vi "黑子权值.vi"(9 "列":u8, 10 "行":dbl, 11 "当前棋盘状态":i32[][](array[numeric])) -> (3 "黑子总权值":i32)   [LabVIEW 2018]
doc: "计算当前位置对于黑子来说的权值大小。"
panel:
  out "活1?右上":bool
  out "活1?左下":bool
  out "活1?左上":bool
  out "活1?右下":bool
  out "活1?正上":bool
  out "活1?正下":bool
  out "活1?正左":bool
  out "活1?正右":bool
  out "3个黑子？右上":bool
  out "2个黑子？右上":bool
  out "1个黑子？右上":bool
  out "3个黑子？左下":bool
  out "2个黑子？左下":bool
  out "1个黑子？ 左下":bool
  out "3个黑子？左上":bool
  out "2个黑子？左上":bool
  out "1个黑子？左上":bool
  out "3个黑子？右下":bool
  out "2个黑子？右下":bool
  out "1个黑子？右下":bool
  out "3个黑子？ 正上":bool
  out "2个黑子？ 正上":bool
  out "1个黑子？ 正上":bool
  out "3个黑子？ 正下":bool
  out "2个黑子？正下":bool
  out "1个黑子？ 正下":bool
  out "3个黑子？正左":bool
  out "2个黑子？正左":bool
  out "1个黑子？正左":bool
  out "3个黑子？正右":bool
  out "2个黑子？正右":bool
  out "1个黑子？正右":bool
  out "右上方向权值":i32
  out "左下方向权值":i32
  out "左上方向权值":i32
  out "右下方向权值":i32
  out "正上方权值":i32
  out "正下方权值":i32
  out "正左方向权值":i32
  out "正右方向权值":i32
  out "前二位权值":dbl
  out "前三位权值":dbl
  # "当前\n位置"
  # "0"
  # "1"
  # "2"
  # "3"
  # "4"
  # "5"
  # "6"
  # "7"
  # "8"
  # "9"
  # "10"
  # "11"
  # "12"
  # "13"
  # "14"
  # "0"
  # "1"
  # "2"
  # "3"
  # "4"
  # "5"
  # "6"
  # "7"
  # "8"
  # "9"
  # "10"
  # "11"
  # "12"
  # "13"
  # "14"
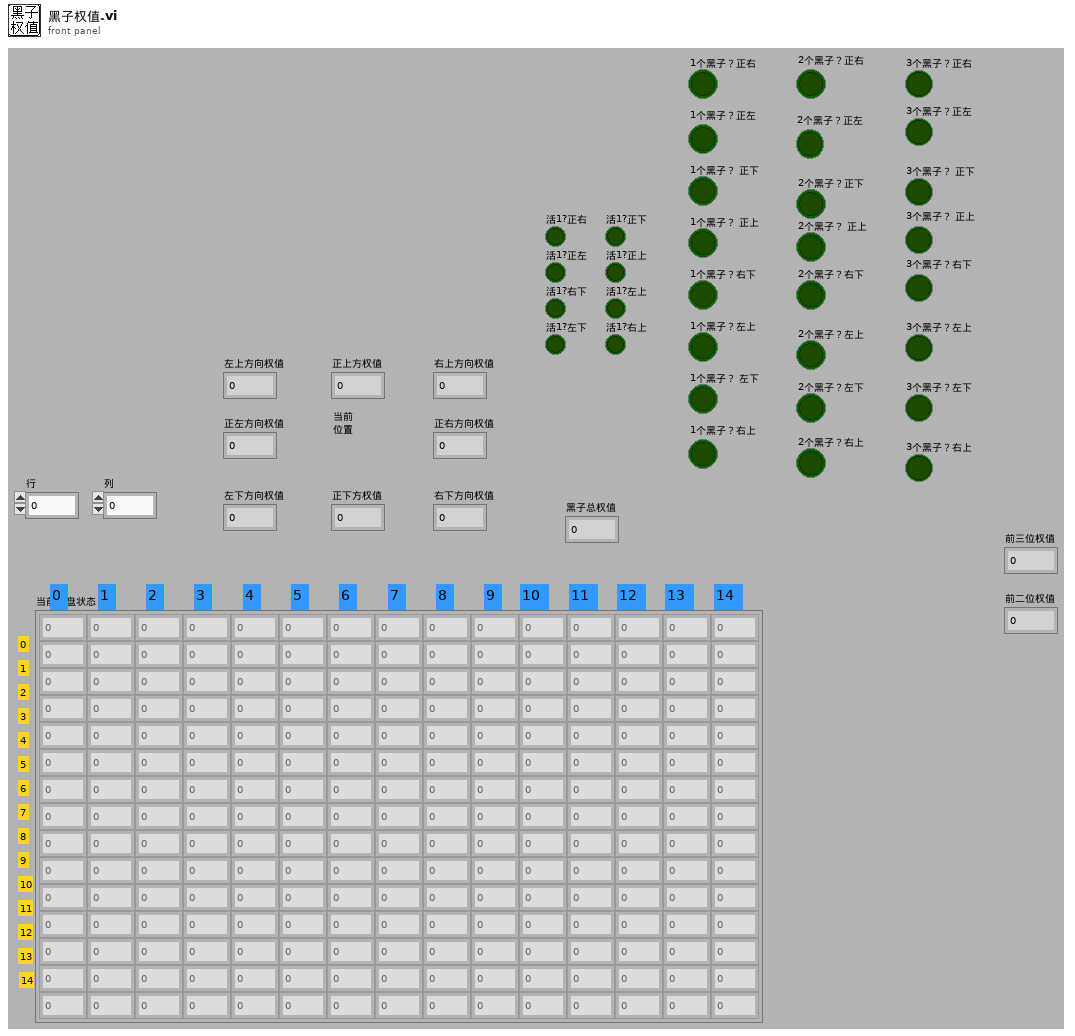
[diagram p1: front panel]
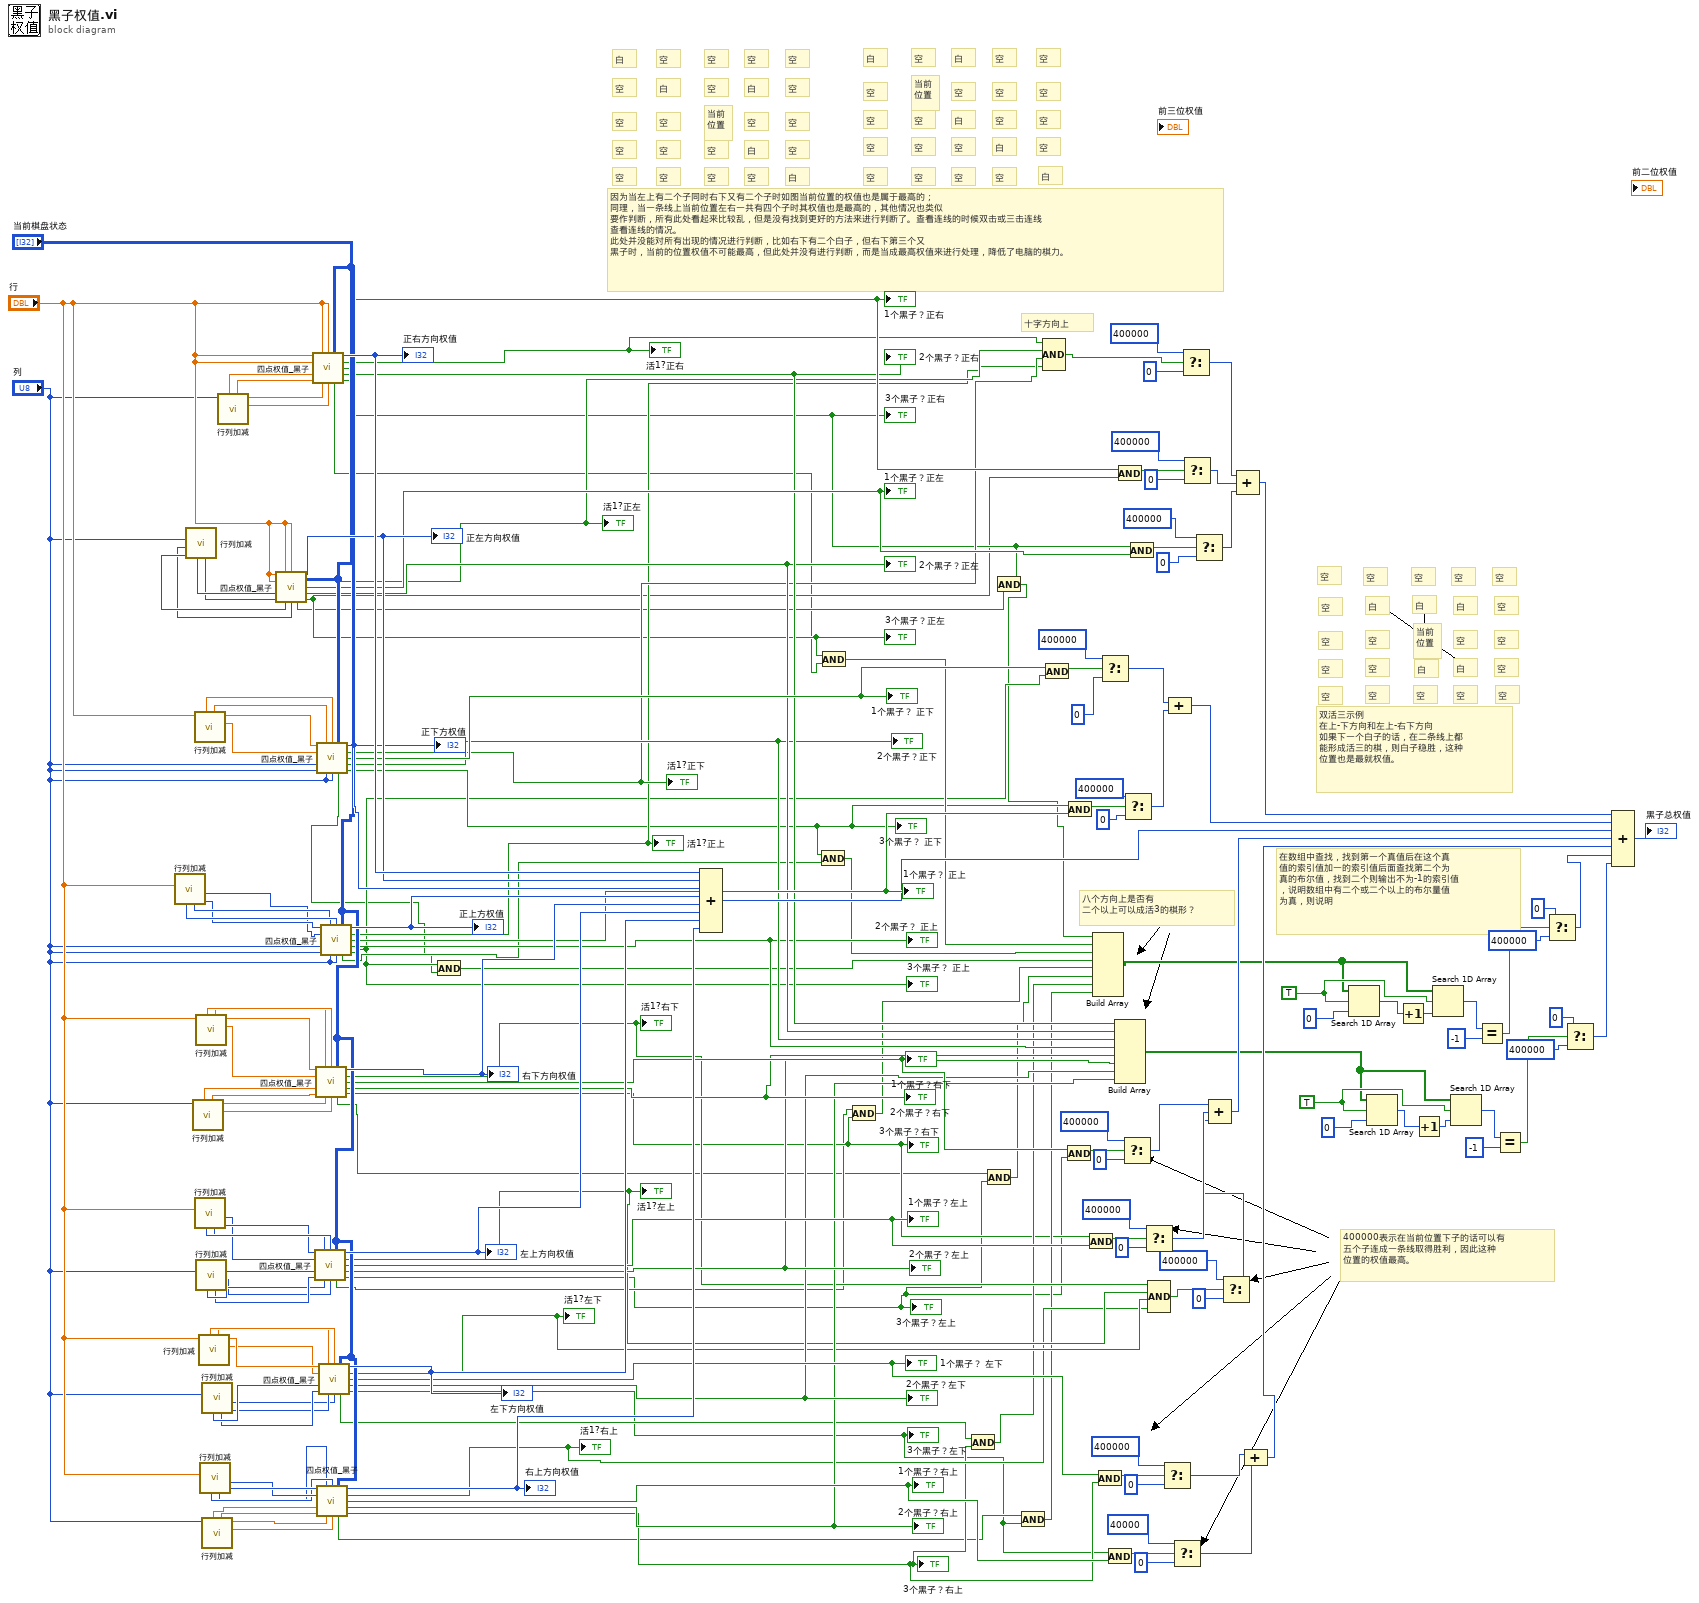
[diagram p0: block diagram]
diagram:
  w48 = TRUE ("element")
  w71 = TRUE ("element")
  # "双活三示例\n在上-下方向和左上-右下方向\n如果下一个白子的话，在二条线上都\n能形成活三的棋，则白子稳胜，这种\n位置也是最就权值。"
  # "空"
  # "空"
  # "空"
  # "空"
  # "空"
  # "空"
  # "空"
  # "空"
  # "空"
  # "空"
  # "空"
  # "空"
  # "空"
  # "空"
  # "空"
  # "空"
  # "空"
  # "白"
  # "白"
  # "白"
  # "白"
  # "空"
  # "白"
  # "空"
  # "当前\n位置"
  # "400000表示在当前位置下子的话可以有\n五个子连成一条线取得胜利，因此这种\n位置的权值最高。"
  # "空"
  # "空"
  # "空"
  # "空"
  # "空"
  # "空"
  # "空"
  # "空"
  # "空"
  # "空"
  # "空"
  # "空"
  # "空"
  # "空"
  # "空"
  # "空"
  # "空"
  # "白"
  # "白"
  # "白"
  # "白"
  # "空"
  # "白"
  # "空"
  # "当前\n位置"
  # "空"
  # "空"
  # "空"
  # "空"
  # "空"
  # "空"
  # "空"
  # "空"
  # "空"
  # "空"
  # "空"
  # "空"
  # "空"
  # "空"
  # "空"
  # "空"
  # "空"
  # "白"
  # "白"
  # "白"
  # "白"
  # "空"
  # "白"
  # "空"
  # "因为当左上有二个子同时右下又有二个子时如图当前位置的权值也是属于最高的；\n同理，当一条线上当前位置左右一共有四个子时其权值也是最高的，其他情况也类似\n要作判断，所有此处看起来比较乱，但是没有找到更好的方法来进行判断了。查看连线的时候双击或三击连线\n查看连线的情况。\n此处并没能对所有出现的情况进行判断，比如右下有二个白子，但右下第三个又\n黑子时，当前的位置权值不可能最高，但此处并没有进行判断，而是当成最高权值来进行处理，降低了电脑的棋力。"
  # "当前\n位置"
  # "十字方向上"
  # "八个方向上是否有\n二个以上可以成活3的棋形？"
  # "在数组中查找，找到第一个真值后在这个真\n值的索引值加一的索引值后面查找第二个为\n真的布尔值，找到二个则输出不为-1的索引值\n，说明数组中有二个或二个以上的布尔量值\n为真，则说明"
  n1 = call "行列加减.vi"("减"="行") -> ("x-3"=w157:i32, "x-4"=w156:i32, "x-2"=w158:i32, "x-1"=w159:i32)  [unwired: 3 in, 4 out]
  n2 = call "行列加减.vi"("减"="列") -> ("x-3"=w165:i32, "x-4"=w164:i32, "x-2"=w166:i32, "x-1"=w167:i32)  [unwired: 3 in, 4 out]
  n3 = call "行列加减.vi"("加"="列") -> ("x+4"=w148:dbl, "x+3"=w149:dbl, "x+2"=w150:dbl, "x+1"=w151:dbl)  [unwired: 3 in, 4 out]
  n4 = call "行列加减.vi"("加"="行") -> ("x+4"=w160:dbl, "x+3"=w161:dbl, "x+2"=w162:dbl, "x+1"=w163:dbl)  [unwired: 3 in, 4 out]
  n5 = call "行列加减.vi"("减"="行") -> ("x-3"=w144:i32, "x-4"=w143:i32, "x-2"=w145:i32, "x-1"=w146:i32)  [unwired: 3 in, 4 out]
  n6 = call "行列加减.vi"("加"="行") -> ("x+4"=w152:dbl, "x+3"=w153:dbl, "x+2"=w154:dbl, "x+1"=w155:dbl)  [unwired: 3 in, 4 out]
  n7 = call "行列加减.vi"("减"="列") -> ("x-3"=w140:i32, "x-4"=w139:i32, "x-2"=w141:i32, "x-1"=w142:i32)  [unwired: 3 in, 4 out]
  n8 = call "行列加减.vi"("加"="行") -> ("x+4"=w134:dbl, "x+3"=w135:dbl, "x+2"=w136:dbl, "x+1"=w137:dbl)  [unwired: 3 in, 4 out]
  n9 = call "行列加减.vi"("减"="行") -> ("x-3"=w125:i32, "x-4"=w124:i32, "x-2"=w117:i32, "x-1"=w118:i32)  [unwired: 3 in, 4 out]
  n10 = call "行列加减.vi"("减"="列") -> ("x-3"=w131:i32, "x-4"=w130:i32, "x-2"=w132:i32, "x-1"=w133:i32)  [unwired: 3 in, 4 out]
  n11 = call "行列加减.vi"("加"="列") -> ("x+4"=w120:dbl, "x+3"=w121:dbl, "x+2"=w122:dbl, "x+1"=w123:dbl)  [unwired: 3 in, 4 out]
  n12 = call "行列加减.vi"("加"="列") -> ("x+4"=w168:dbl, "x+3"=w169:dbl, "x+2"=w170:dbl, "x+1"=w171:dbl)  [unwired: 3 in, 4 out]
  n13 = call "四点权值_黑子.vi"("3位置行"="行", "2位置行"="行", "1位置行"="行", "当前棋盘状态"="当前棋盘状态", "4位置行"="行", "1位置列"=w167, "2位置列"=w166, "3位置列"=w165, "4位置列"=w164) -> ("黑子四位置权值"=w174:i32, "有2个黑子?或黑子加无子?"=w39:bool, "第1个位置是黑子?"=w108:bool, "3个黑子?"=w60:bool, "第一个位置为空"=w19:bool, "3个黑子？或2个黑子加无子?"=w23:bool)  [unwired: 1 in]
  "正左方向权值" <- w174
  "1个黑子？正左" <- w108
  "2个黑子？正左" <- w60
  "3个黑子？正左" <- w23
  "活1?正左" <- w39
  n14 = call "四点权值_黑子.vi"("3位置行"="行", "2位置行"="行", "1位置行"="行", "当前棋盘状态"="当前棋盘状态", "4位置行"="行", "1位置列"=w171, "2位置列"=w170, "3位置列"=w169, "4位置列"=w168) -> ("黑子四位置权值"=w175:i32, "有2个黑子?或黑子加无子?"=w40:bool, "第1个位置是黑子?"=w112:bool, "3个黑子?"=w61:bool, "第一个位置为空"=w18:bool, "3个黑子？或2个黑子加无子?"=w24:bool)  [unwired: 1 in]
  "正右方向权值" <- w175
  "1个黑子？正右" <- w112
  "2个黑子？正右" <- w61
  "3个黑子？正右" <- w24
  "活1?正右" <- w40
  n15 = call "四点权值_黑子.vi"("3位置行"=w144, "2位置行"=w145, "1位置行"=w146, "当前棋盘状态"="当前棋盘状态", "4位置行"=w143, "1位置列"=w142, "2位置列"=w141, "3位置列"=w140, "4位置列"=w139) -> ("黑子四位置权值"=w138:i32, "有2个黑子?或黑子加无子?"=w31:bool, "第1个位置是黑子?"=w86:bool, "3个黑子?"=w56:bool, "第一个位置为空"=w7:bool, "3个黑子？或2个黑子加无子?"=w5:bool)  [unwired: 1 in]
  "左上方向权值" <- w138
  "1个黑子？左上" <- w86
  "2个黑子？左上" <- w56
  "3个黑子？左上" <- w5
  "活1?左上" <- w31
  n16 = call "四点权值_黑子.vi"("3位置行"=w153, "2位置行"=w154, "1位置行"=w155, "当前棋盘状态"="当前棋盘状态", "4位置行"=w152, "1位置列"=w151, "2位置列"=w150, "3位置列"=w149, "4位置列"=w148) -> ("黑子四位置权值"=w147:i32, "有2个黑子?或黑子加无子?"=w32:bool, "第1个位置是黑子?"=w91:bool, "3个黑子?"=w57:bool, "第一个位置为空"=w6:bool, "3个黑子？或2个黑子加无子?"=w8:bool)  [unwired: 1 in]
  "右下方向权值" <- w147
  "1个黑子？右下" <- w91
  "2个黑子？右下" <- w57
  "3个黑子？右下" <- w8
  "活1?右下" <- w32
  n17 = call "四点权值_黑子.vi"("3位置行"=w161, "2位置行"=w162, "1位置行"=w163, "当前棋盘状态"="当前棋盘状态", "4位置行"=w160, "1位置列"="列", "2位置列"="列", "3位置列"="列", "4位置列"="列") -> ("黑子四位置权值"=w173:i32, "有2个黑子?或黑子加无子?"=w38:bool, "第1个位置是黑子?"=w102:bool, "3个黑子?"=w59:bool, "第一个位置为空"=w15:bool, "3个黑子？或2个黑子加无子?"=w20:bool)  [unwired: 1 in]
  "正下方权值" <- w173
  "1个黑子？ 正下" <- w102
  "2个黑子？正下" <- w59
  "3个黑子？ 正下" <- w20
  "活1?正下" <- w38
  n18 = call "四点权值_黑子.vi"("3位置行"=w125, "2位置行"=w117, "1位置行"=w118, "当前棋盘状态"="当前棋盘状态", "4位置行"=w124, "1位置列"=w123, "2位置列"=w122, "3位置列"=w121, "4位置列"=w120) -> ("黑子四位置权值"=w119:i32, "有2个黑子?或黑子加无子?"=w29:bool, "第1个位置是黑子?"=w74:bool, "3个黑子?"=w54:bool, "第一个位置为空"=w2:bool, "3个黑子？或2个黑子加无子?"=w3:bool)  [unwired: 1 in]
  "右上方向权值" <- w119
  "1个黑子？右上" <- w74
  "2个黑子？右上" <- w54
  "3个黑子？右上" <- w3
  "活1?右上" <- w29
  n19 = call "四点权值_黑子.vi"("3位置行"=w135, "2位置行"=w136, "1位置行"=w137, "当前棋盘状态"="当前棋盘状态", "4位置行"=w134, "1位置列"=w133, "2位置列"=w132, "3位置列"=w131, "4位置列"=w130) -> ("黑子四位置权值"=w129:i32, "有2个黑子?或黑子加无子?"=w30:bool, "第1个位置是黑子?"=w79:bool, "3个黑子?"=w55:bool, "第一个位置为空"=w4:bool, "3个黑子？或2个黑子加无子?"=w1:bool)  [unwired: 1 in]
  "左下方向权值" <- w129
  "1个黑子？ 左下" <- w79
  "2个黑子？左下" <- w55
  "3个黑子？左下" <- w1
  "活1?左下" <- w30
  n20 = call "四点权值_黑子.vi"("3位置行"=w157, "2位置行"=w158, "1位置行"=w159, "当前棋盘状态"="当前棋盘状态", "4位置行"=w156, "1位置列"="列", "2位置列"="列", "3位置列"="列", "4位置列"="列") -> ("黑子四位置权值"=w172:i32, "有2个黑子?或黑子加无子?"=w37:bool, "第1个位置是黑子?"=w98:bool, "3个黑子?"=w58:bool, "第一个位置为空"=w17:bool, "3个黑子？或2个黑子加无子?"=w16:bool)  [unwired: 1 in]
  "正上方权值" <- w172
  "1个黑子？ 正上" <- w98
  "2个黑子？ 正上" <- w58
  "3个黑子？ 正上" <- w16
  "活1?正上" <- w37
  n21 = And(x=w16, y=w15) -> (x .and. y?=w14:bool)
  n22 = Compound Arithmetic op=ADD(w175, w174, w173, w172, w147, w138, w129, w119) -> (w95:i32)
  n23 = And(x=w20, y=w17) -> (x .and. y?=w21:bool)
  n24 = And(x=w23, y=w18) -> (x .and. y?=w22:bool)
  n25 = And(x=w7, y=w8) -> (x .and. y?=w13:bool)
  n26 = And(x=w4, y=w3) -> (x .and. y?=w11:bool)
  n27 = And(x=w6, y=w5) -> (x .and. y?=w12:bool)
  n28 = And(x=w24, y=w19) -> (x .and. y?=w9:bool)
  n29 = And(x=w2, y=w1) -> (x .and. y?=w10:bool)
  n30 = And(x=w102, y=w16) -> (x .and. y?=w105:bool)
  n31 = Compound Arithmetic op=AND(w40, w39, w38, w37) -> (w34:bool)
  n32 = And(x=w91, y=w5) -> (x .and. y?=w92:bool)
  n33 = And(x=w20, y=w98) -> (x .and. y?=w101:bool)
  n34 = And(x=w8, y=w86) -> (x .and. y?=w89:bool)
  n35 = Build Array(w9, w22, w21, w14, w13, w12, w11, w10) -> (w68:bool[])
  n36 = And(x=w79, y=w3) -> (x .and. y?=w83:bool)
  n37 = Select(t=400000, s=w105, f=0) -> (s? t:f=w62:i32)
  n38 = And(x=w1, y=w74) -> (x .and. y?=w75:bool)
  n39 = And(x=w112, y=w23) -> (x .and. y?=w114:bool)
  n40 = Build Array(w61, w60, w59, w58, w57, w56, w55, w54) -> (w46:bool[])
  n41 = Select(t=400000, s=w92, f=0) -> (s? t:f=w90:i32)
  n42 = Select(t=400000, s=w101, f=0) -> (s? t:f=w97:i32)
  n43 = And(x=w24, y=w108) -> (x .and. y?=w111:bool)
  n44 = Select(t=400000, s=w89, f=0) -> (s? t:f=w85:i32)
  n45 = Compound Arithmetic op=AND(w32, w31, w30, w29) -> (w27:bool)
  n46 = Select(t=400000, s=w83, f=0) -> (s? t:f=w78:i32)
  n47 = Compound Arithmetic op=ADD(w62, w97) -> (w96:i32)
  n48 = Select(t=40000, s=w75, f=0) -> (s? t:f=w73:i32)
  n49 = Select(t=400000, s=w34, f=0) -> (s? t:f=w33:i32)
  n50 = Select(t=400000, s=w114, f=0) -> (s? t:f=w113:i32)
  n51 = Select(t=400000, s=w111, f=0) -> (s? t:f=w107:i32)
  n52 = Select(t=400000, s=w27, f=0) -> (s? t:f=w25:i32)
  n53 = Compound Arithmetic op=ADD(w90, w85, w25) -> (w84:i32)
  n54 = Compound Arithmetic op=ADD(w33, w113, w107) -> (w106:i32)
  n55 = Compound Arithmetic op=ADD(w78, w73) -> (w80:i32)
  n56 = Search 1D Array(1D array=w68, element=w71, start index (0)=0) -> (index of element=w43:i32)
  n57 = Search 1D Array(1D array=w46, element=w48, start index (0)=0) -> (index of element=w41:i32)
  n58 = Increment(x=w43) -> (x+1=w44:i32)
  n59 = Increment(x=w41) -> (x+1=w42:i32)
  n60 = Search 1D Array(1D array=w68, element=w71, start index (0)=w44) -> (index of element=w70:i32)
  n61 = Search 1D Array(1D array=w46, element=w48, start index (0)=w42) -> (index of element=w49:i32)
  n62 = Equal?(x=w70, y=-1) -> (x = y?=w66:bool)
  n63 = Equal?(x=w49, y=-1) -> (x = y?=w52:bool)
  n64 = Select(t=0, s=w66, f=400000) -> (s? t:f=w65:i32)
  n65 = Select(t=0, s=w52, f=400000) -> (s? t:f=w45:i32)
  n66 = Compound Arithmetic op=ADD(w106, w96, w95, w84, w80, w65, w45) -> (→"黑子总权值":i32)
